vi "S2C_5190CR_Proc_CacheState.vi"(7 "Label":string, 8 "Error In":errorcluster, 10 "Command":string, 11 "Data In":string) -> (0 "Error Out":errorcluster, 3 "Data Out":string)   [LabVIEW 2015]
doc: "Updates the front panel controls based on the data passed in."
uses:
  S2C_5190CR_Proc_Globals.vi
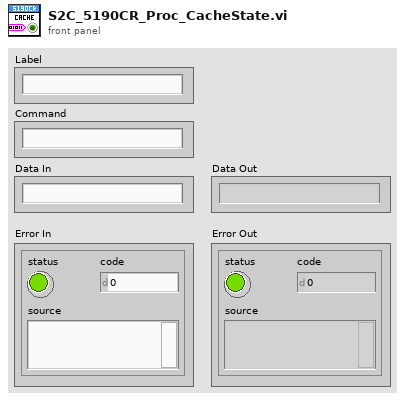
[diagram p1: front panel]
types:
  T1 = cluster{"IP Address":string, "Port":u16, "Username":string, "Password":string, "Timeout(ms)":i32, "P1C1Exe":bool}
  T2 = cluster{"IP Address":string, "Port":u16, "Username":string, "Password":string, "Timeout(ms)":i32}
  T3 = cluster{"Command":u16, "OutletPlug":u16, "Current":string, "Power":string, "Voltage":string, "Timeout(ms)":u32, "P1C2Exe":bool}
  T4 = cluster{"OutletPlug":u16, "OutletState":bool, "PowerOnDelay(ms)":u32, "PowerOffDelay(ms)":u32, "WaitOnState":bool, "Timeout(ms)":i32, "P1C3Exe":bool}
  T5 = cluster{"OutletPlug":u16, "OutletState":bool, "PowerOnDelay(ms)":u32, "PowerOffDelay(ms)":u32, "WaitOnState":bool, "Timeout(ms)":i32}
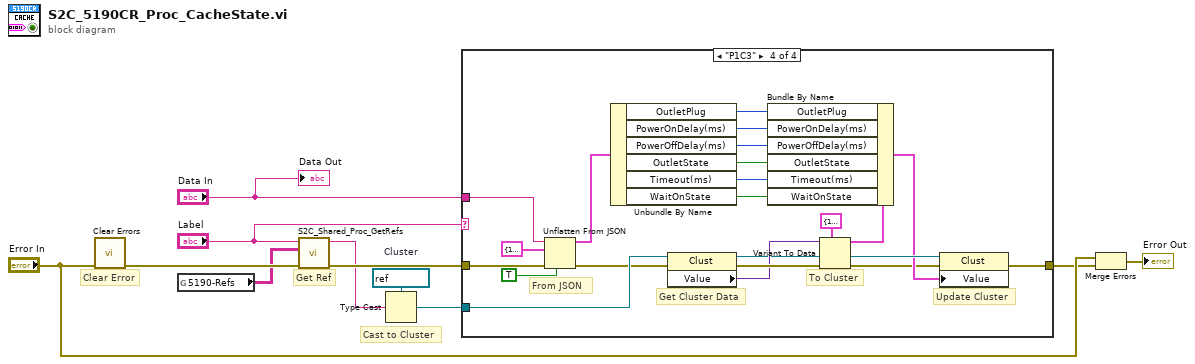
[diagram p0: block diagram]
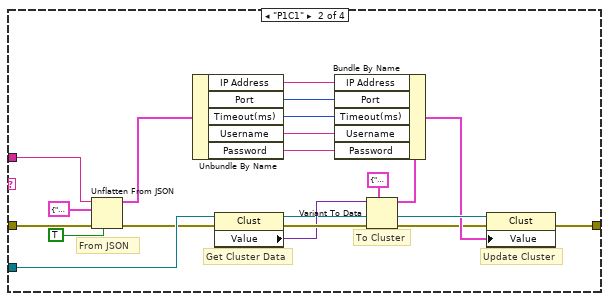
[diagram p3: hidden frame]
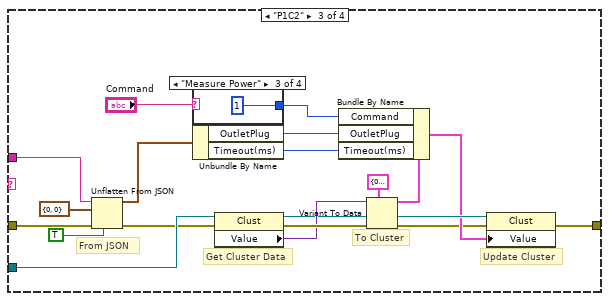
[diagram p4: hidden frame]
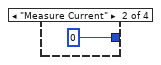
[diagram p6: hidden frame]
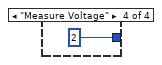
[diagram p7: hidden frame]
diagram:
  w7 = refnum<vi> refnum  # Cluster
  # "Cast to Cluster"
  # "Get Ref"
  # "Clear Error"
  n1 = call <vilib>:"Clear Errors.vi"("error in (no error)"="Error In") -> ("error out"=w4:errorcluster)  [unwired: 5 in, 1 out]
  n2 = global read "S2C_5190CR_Proc_Globals.vi" "5190-Refs"() -> (w1:string[][])
  n3 = call "S2C_Shared_Proc_GetRefs.vi"("Error In"=w4, "Refs"=w1, "Label"="Label") -> ("Error Out"=w9:errorcluster, "Reference"=w6:string)  [unwired: 7 in]
  n4 = Type Cast(type=w7, x=w6) -> (*(type *) &x=w5:refnum<vi>)
  n5 = case shown="\"P1C3\"" "Label" {
    tunnel: w9 -> [w12 w24 w45 w70]
    tunnel: [w12 w18 w39 w64] -> w2
    tunnel: w5 -> [_ w26 w47 w72]
    tunnel: "Data In" -> [_ w22 w43 w68]
    frame "Other", Default {
    }
    frame "P1C1" {
      # "Update Cluster"
      # "To Cluster"
      # "Get Cluster Data"
      # "From JSON"
      n6 = Unflatten From JSON(JSON string=w22, type and defaults=T2 {"IP Address"="", "Port"=57600, "Username"="", "Password"="", "Timeout(ms)"=5000} ("P1C1"), default null elements? (F)=TRUE, error in (no error)=w24) -> (value=w23:T2, error out=w21:errorcluster)  [unwired: 3 in]
      n7 = Unbundle By Name(w23) -> ("IP Address"=w29:string, "Port"=w28:u16, "Timeout(ms)"=w27:i32, "Username"=w16:string, "Password"=w15:string)
      n8 = property class="Clust"(reference=w26, error in=w21) -> (reference out=w20:refnum<vi>, error out=w32:errorcluster, "Value"=w31:variant)
      n9 = Variant To Data(error in=w32, type=T1 {"IP Address"="", "Port"=57600, "Username"="", "Password"="", "Timeout(ms)"=5000, "P1C1Exe"=FALSE} ("P1C1"), Variant=w31) -> (data=w30:T1, error out=w17:errorcluster)
      n10 = Bundle By Name(cluster=w30, "IP Address"=w29, "Port"=w28, "Timeout(ms)"=w27, "Username"=w16, "Password"=w15) -> (w19:T1)
      n11 = property class="Clust"(reference=w20, error in=w17, "Value"=w19) -> (error out=w18:errorcluster)  [unwired: 1 out]
    }
    frame "P1C2" {
      # "Update Cluster"
      # "To Cluster"
      # "Get Cluster Data"
      # "From JSON"
      n12 = Unflatten From JSON(JSON string=w43, type and defaults=cluster{"OutletPlug":u16, "Timeout(ms)":i32} {"OutletPlug"=0, "Timeout(ms)"=0} ("P1C2"), default null elements? (F)=TRUE, error in (no error)=w45) -> (value=w44:cluster{"OutletPlug":u16, "Timeout(ms)":i32}, error out=w42:errorcluster)  [unwired: 3 in]
      n13 = case shown="\"Measure Power\"" "Command" {
        tunnel: [_ u16 0 ("Command") u16 1 ("Command") u16 2 ("Command")] -> w33
        frame "Other", Default {
        }
        frame "Measure Current" {
        }
        frame "Measure Power" {
        }
        frame "Measure Voltage" {
        }
      }
      n14 = Unbundle By Name(w44) -> ("OutletPlug"=w48:u16, "Timeout(ms)"=w35:i32)
      n15 = property class="Clust"(reference=w47, error in=w42) -> (reference out=w41:refnum<vi>, error out=w51:errorcluster, "Value"=w50:variant)
      n16 = Variant To Data(error in=w51, type=T3 {"Command"=0, "OutletPlug"=0, "Current"="", "Power"="", "Voltage"="", "Timeout(ms)"=0, "P1C2Exe"=FALSE} ("P1C2"), Variant=w50) -> (data=w49:T3, error out=w38:errorcluster)
      n17 = Bundle By Name(cluster=w49, "Command"=w33, "OutletPlug"=w48, "Timeout(ms)"=w35) -> (w40:T3)
      n18 = property class="Clust"(reference=w41, error in=w38, "Value"=w40) -> (error out=w39:errorcluster)  [unwired: 1 out]
    }
    frame "P1C3" {
      # "Update Cluster"
      # "To Cluster"
      # "Get Cluster Data"
      # "From JSON"
      n19 = Unflatten From JSON(JSON string=w68, type and defaults=T5 {"OutletPlug"=1, "OutletState"=TRUE, "PowerOnDelay(ms)"=50, "PowerOffDelay(ms)"=0, "WaitOnState"=TRUE, "Timeout(ms)"=10000} ("P1C3"), default null elements? (F)=TRUE, error in (no error)=w70) -> (value=w69:T5, error out=w67:errorcluster)  [unwired: 3 in]
      n20 = Unbundle By Name(w69) -> ("OutletPlug"=w62:u16, "PowerOnDelay(ms)"=w57:u32, "PowerOffDelay(ms)"=w58:u32, "OutletState"=w59:bool, "Timeout(ms)"=w60:i32, "WaitOnState"=w61:bool)
      n21 = property class="Clust"(reference=w72, error in=w67) -> (reference out=w66:refnum<vi>, error out=w75:errorcluster, "Value"=w74:variant)
      n22 = Variant To Data(error in=w75, type=T4 {"OutletPlug"=1, "OutletState"=TRUE, "PowerOnDelay(ms)"=50, "PowerOffDelay(ms)"=0, "WaitOnState"=TRUE, "Timeout(ms)"=10000, "P1C3Exe"=FALSE} ("P1C3"), Variant=w74) -> (data=w73:T4, error out=w63:errorcluster)
      n23 = Bundle By Name(cluster=w73, "OutletPlug"=w62, "PowerOnDelay(ms)"=w57, "PowerOffDelay(ms)"=w58, "OutletState"=w59, "Timeout(ms)"=w60, "WaitOnState"=w61) -> (w65:T4)
      n24 = property class="Clust"(reference=w66, error in=w63, "Value"=w65) -> (error out=w64:errorcluster)  [unwired: 1 out]
    }
  }
  n25 = Merge Errors("Error In", w2) -> (→"Error Out":errorcluster)
  "Data Out" <- "Data In"
